vi "Draw.vi"(8 "error in (no error)":errorcluster, 10 "2D Picture in":picture, 11 "Circle in":refnum<class "Circle.lvclass">) -> (0 "error out":errorcluster, 2 "2D Picture out":picture, 3 "Circle out":refnum<class "Circle.lvclass">)   [LabVIEW 2021, in "Picture2D.lvlib" / "Circle.lvclass"]
uses:
  Circle.lvclass
  Circle.lvclass/Circle.ctl
  Color/Color.lvclass
  Point/Point.lvclass
  Pen/Pen.lvclass
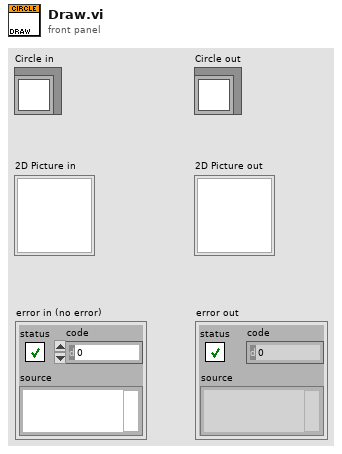
[diagram p1: front panel]
types:
  T1 = cluster{"Width":u16, "Style":enum32{"Solid", "Dash", "Dot", "DashDot", "DashDotDot"}}
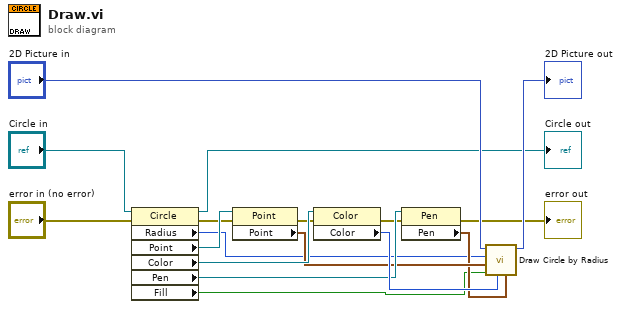
[diagram p0: block diagram]
diagram:
  n1 = property class="Circle"(reference="Circle in", error in="error in (no error)") -> (reference out=→"Circle out":refnum<class "Circle.lvclass">, error out=w6:errorcluster, "Radius"=w7:i16, "Point"=w8:refnum<class "Point.lvclass">, "Color"=w15:refnum<class "Color.lvclass">, "Pen"=w13:refnum<class "Pen.lvclass">, "Fill"=w1:bool)
  n2 = property class="Point"(reference=w8, error in=w6) -> (error out=w5:errorcluster, "Point"=w10:cluster{"x":i16, "y":i16})  [unwired: 1 out]
  n3 = property class="Color"(reference=w15, error in=w5) -> (error out=w4:errorcluster, "Color"=w14:u32)  [unwired: 1 out]
  n4 = property class="Pen"(reference=w13, error in=w4) -> (error out=→"error out":errorcluster, "Pen"=w9:T1)  [unwired: 1 out]
  n5 = call <vilib>:"Draw Circle by Radius.vi"("pen"=w9, "color(black)"=w14, "fill?(F)"=w1, "pixel center"=w10, "radius"=w7, "picture"="2D Picture in") -> ("new picture"=→"2D Picture out":picture)  [unwired: 5 in]
